vi "Bang Bang Temperature Controller.vi"() -> ()   [LabVIEW 2021]
uses:
  BT.lvlib
  Support/Nodes/Decorators/Repeater/Support/Finish On - Type.ctl
  Support/Nodes/Decorators/Repeater/bt_Repeater.lvclass
  <vilib>/TSA/Omni-Bus/Omni-Bus/Omni_Bus.lvclass
  <vilib>/TSA/Abstract Data Classes/Constants/Support/DBL/DBL.vi
  <vilib>/TSA/Abstract Data Classes/Constants/Support/DBL/Const_DBL.lvclass
  C:/Program Files (x86)/National Instruments/LabVIEW 2021/vi.lib/TSA/Abstract Data Classes/Abs_Types/Double Float/Abs_Double Float.lvclass
  C:/Program Files (x86)/National Instruments/LabVIEW 2021/vi.lib/TSA/Abstract Data Classes/Abs_Types/Floating Point/Abs_Floating Point.lvclass
  C:/Program Files (x86)/National Instruments/LabVIEW 2021/vi.lib/TSA/Abstract Data Classes/Abs_Types/Numeric/Abs_Numeric.lvclass
  C:/Program Files (x86)/National Instruments/LabVIEW 2021/vi.lib/TSA/Abstract Data Classes/Abs_Types/Value/Abs_Value.lvclass
  C:/Program Files (x86)/National Instruments/LabVIEW 2021/vi.lib/TSA/Abstract Data Classes/Abs_Types/Type/Abs_Type.lvclass
  C:/Program Files (x86)/National Instruments/LabVIEW 2021/vi.lib/TSA/Abstract Data Classes/Constants/Support/DBL/Const_DBL.lvclass
  C:/Program Files (x86)/National Instruments/LabVIEW 2021/vi.lib/TSA/Abstract Data Classes/Constants/Support/Interface/Const_Intf.lvclass
  <vilib>/TSA/Omni-Bus/Local Bus/Local Bus.lvclass
  <vilib>/Utility/Data Type/Type Definitions/Data Type.ctl
  <vilib>/Utility/Data Type/NI_Data Type.lvlib
  <vilib>/TSA/Omni-Bus/Local Bus/Support/Tag List Type.ctl
  System/bt_System.lvclass
  <vilib>/TSA/Omni-Bus/Omni-Bus/Support/Get/Get DBL.vi
  <vilib>/TSA/Omni-Bus/Omni-Bus/Support/Get/Get Boolean.vi
  <vilib>/TSA/Omni-Bus/Omni-Bus/Support/Read/Read Boolean.vi
  <vilib>/TSA/Omni-Bus/Omni-Bus/Support/Write/Write DBL.vi
  <vilib>/TSA/Event Log/abs_EventLog/Support/Facility Code.ctl
  <vilib>/TSA/Event Log/abs_EventLog/abs_EventLog.lvclass
  <vilib>/TSA/Event Log/abs_EventLog/Support/Severity Code.ctl
  <vilib>/TSA/Event Log/Event_TextLog/Event_TextLog.lvclass
  C:/Program Files (x86)/National Instruments/LabVIEW 2021/vi.lib/TSA/Omni-Bus/Omni-Bus/Bus Access/Bus_Access.lvclass
  C:/Program Files (x86)/National Instruments/LabVIEW 2021/vi.lib/TSA/Omni-Bus/Local Bus/Local Bus.lvclass
  C:/Program Files (x86)/National Instruments/LabVIEW 2021/vi.lib/TSA/Event Log/abs_EventLog/abs_EventLog.lvclass
  C:/Program Files (x86)/National Instruments/LabVIEW 2021/vi.lib/TSA/Event Log/Event_TextLog/Event_TextLog.lvclass
  Support/Nodes/abs_Node/Status.ctl
  Support/Nodes/abs_Node/bt_Node.lvclass
panel:
  out "Event Messages":string
  out "Status":T1
  out "Waveform Chart":cluster{"Temperature Reading":dbl, i16}(graph)
  in  "stop":bool
  in  "Temperature Reading\n(User Simulated)":dbl(slide) scale=0.0..100.0
  out "Heater":bool
  in  "Hystersis":dbl=2.0
  in  "Temperature Setting":dbl=50.0
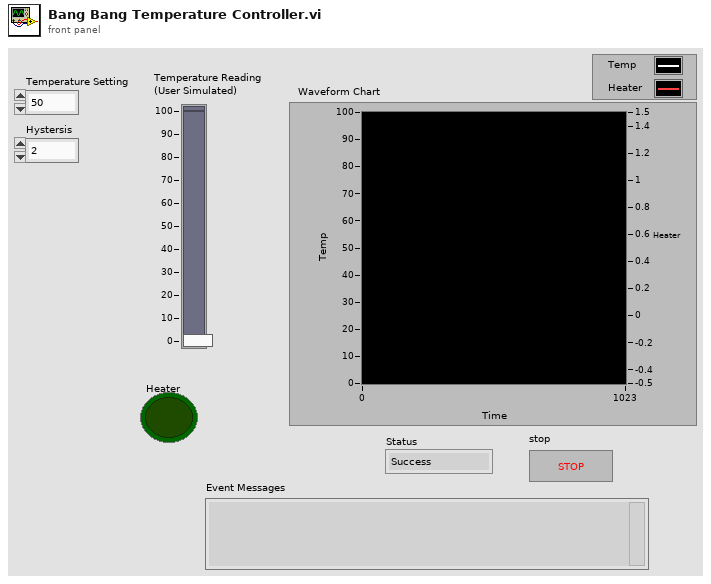
[diagram p1: front panel]
types:
  T1 = typedef "BT.lvlib/bt_Node.lvclass/Status.ctl" = enum16{"Success", "Failure", "Running"}
  T2 = typedef "abs_EventLog.lvclass/Severity Code.ctl" = enum16{"emergency", "alert", "critical", "error", "warning", "notice", "info", "debug"}
  T3 = typedef "abs_EventLog.lvclass/Facility Code.ctl" = enum16{"kernel", "user", "mail", "system daemons", "security/authorization", "syslogd", "line printer", "network news", "uucp", "clock daemon", "security/authorization (alternate)", "FTP daemon", "NTP subsystem", "log audit", "log alert", "clock daemon (alternate)", "local use 0", "local use 1", "local use 2", "local use 3", "local use 4", "local use 5", "local use 6", "local use 7"}
  T4 = typedef "Local Bus.lvclass/Tag List Type.ctl" = cluster{"Tag":string, "Type":T5}
  T5 = typedef "NI_Data Type.lvlib/Data Type.ctl" = enum8{"Invalid Type", "Void", "I8", "I16", "I32", "I64", "U8", "U16", "U32", "U64", "Single Float", "Double Float", "Extended Float", "Single Complex", "Double Complex", "Extended Complex", "Enum U8", "Enum U16", "Enum U32", "Enum U64", "Single Float With Unit", "Double Float With Unit", "Extended Float With Unit", "Single Complex with Unit", "Double Complex with Unit", "Extended Complex with Unit", "Boolean", "String", "Path", "Picture", "Tag", "Array", "Cluster", "Variant", "LV Variant", "Waveform", "Timestamp", "Digital Waveform", "Digital Data", "ExpressData", "Refnum", "External Data", "VI", "Poly VI", "LabVIEW Class Instance", "Fixed Point", "Set Collection", "Map Collection"}
  T6 = typedef "BT.lvlib/bt_Repeater.lvclass/Finish On - Type.ctl" = enum16{"Success", "Failure", "Never"}
  T7 = cluster{"Temperature Reading\n(User Simulated)":dbl, i16}
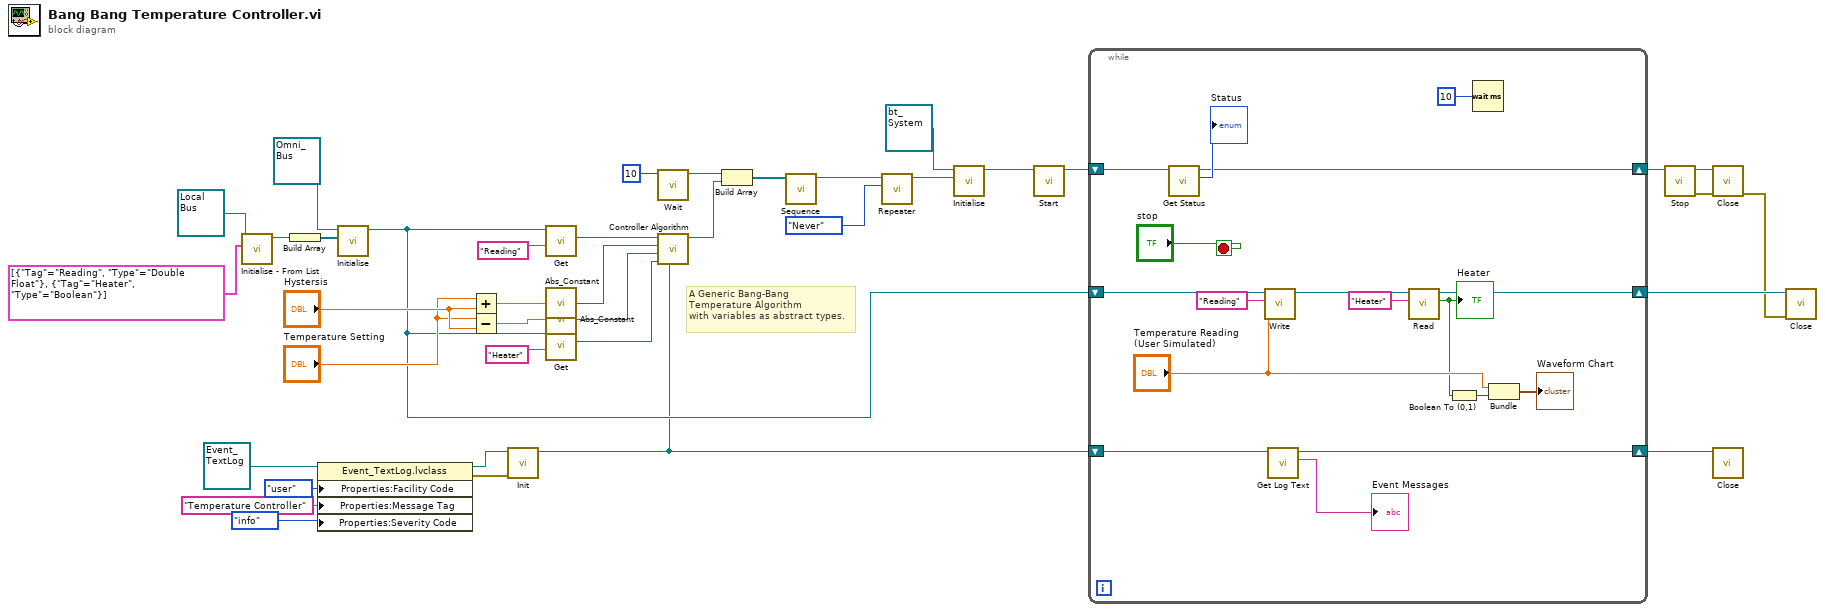
[diagram p0: block diagram]
diagram:
  # "A Generic Bang-Bang \nTemperature Algorithm\nwith variables as abstract types."
  n1 = call <vilib>:"Initialise - From List.vi"("Tag List"=T4[] [{"Tag"="Reading", "Type"=enum."Double Float"}, {"Tag"="Heater", "Type"=enum."Boolean"}], "Local Bus in"=refnum<class "Local Bus.lvclass"> refnum) -> ("Local Bus out"=w21:refnum<class "Local Bus.lvclass">)  [unwired: 8 in, 1 out]
  n2 = Build Array(w21) -> (w22:refnum<class "Local Bus.lvclass">[])
  n3 = property class="Event_TextLog.lvclass"(reference=refnum<class "Event_TextLog.lvclass"> refnum ("Event_TextLog.lvclass"), "Properties:Facility Code"=Facility_Code."user" ("Facility Code"), "Properties:Message Tag"="Temperature Controller" ("Message Tag"), "Properties:Severity Code"=Severity_Code."info" ("Severity Code")) -> (reference out=w3:refnum<class "Event_TextLog.lvclass">, error out=w2:errorcluster)  [unwired: 1 in]
  n4 = call-dynamic "Initialise.vi"("Bus Access"=w22, "Var Bus in"=refnum<class "Omni_Bus.lvclass"> refnum) -> ("Var Bus out"=w19:refnum<class "Omni_Bus.lvclass">)  [unwired: 8 in, 1 out]
  n5 = Add(x="Temperature Setting", y="Hystersis") -> (x+y=w32:dbl)
  n6 = Subtract(x="Temperature Setting", y="Hystersis") -> (x-y=w31:dbl)
  n7 = call-dynamic "Init.vi"("error in (no error)"=w2, "Event_TextLog in"=w3) -> ("Event_TextLog out"=w1:refnum<class "Event_TextLog.lvclass">)  [unwired: 8 in, 1 out]
  n8 = call-poly <vilib>:"Get.vi"("Tag"="Reading", "Var Bus in"=w19) -> ("Value Out"=w38:refnum<class "Abs_Double Float.lvclass">)  [unwired: 6 in, 3 out]
  n9 = call-poly <vilib>:"Abs_Constant.vi"("Value"=w32) -> ("Constant"=w37:refnum<class "Const_DBL.lvclass">)  [unwired: 4 in]
  n10 = call-poly <vilib>:"Abs_Constant.vi"("Value"=w31) -> ("Constant"=w36:refnum<class "Const_DBL.lvclass">)  [unwired: 4 in]
  n11 = call-poly <vilib>:"Get.vi"("Tag"="Heater", "Var Bus in"=w19) -> ("Value Out"=w35:refnum<class "Abs_Boolean.lvclass">)  [unwired: 6 in, 3 out]
  n12 = call "Wait.vi"("Time (ms)"=u32 10) -> ("Node Out"=w26:refnum<class "bt_Node.lvclass">)  [unwired: 10 in]
  n13 = call "Controller Algorithm.vi"("EventLog"=w1, "Heater Output"=w35, "Lower Limit"=w36, "Upper Limit"=w37, "Reading"=w38) -> ("Node Out"=w28:refnum<class "bt_Node.lvclass">)  [unwired: 6 in]
  n14 = Build Array(w26, w28) -> (w27:refnum<class "bt_Node.lvclass">[])
  n15 = call "Sequence.vi"("Nodes"=w27) -> ("Node"=w24:refnum<class "bt_Node.lvclass">)  [unwired: 10 in]
  n16 = call "Repeater.vi"("Finish On"=Finish_On_-_Type."Never", "Node In"=w24) -> ("Node Out"=w10:refnum<class "bt_Node.lvclass">)  [unwired: 9 in]
  n17 = call "Initialise.vi"("Behaviour Tree"=w10, "bt_System in"=refnum<class "bt_System.lvclass"> refnum) -> ("bt_System out"=w11:refnum<class "bt_System.lvclass">)  [unwired: 8 in, 1 out]
  n18 = call "Start.vi"("bt_System in"=w11) -> ("bt_System out"=w15:refnum<class "bt_System.lvclass">)  [unwired: 9 in, 1 out]
  n19 = while {
    shift-right: [w43] -> w14
    shift-left: w15 -> [w46]
    shift-right: [w54] -> w17
    shift-left: w19 -> [w56]
    shift-right: [w41] -> w4
    shift-left: w1 -> [w42]
    stop <- "stop" stop-if-true
    n20 = call "Get Status.vi"("bt_System in"=w46) -> ("Status"=→"Status":T1, "bt_System out"=w43:refnum<class "bt_System.lvclass">)  [unwired: 8 in, 1 out]
    n21 = call-poly <vilib>:"Write.vi"("Numeric"="Temperature Reading\n(User Simulated)", "Tag"="Reading", "Omni_Bus in"=w56) -> ("Omni_Bus out"=w55:refnum<class "Omni_Bus.lvclass">)  [unwired: 7 in, 1 out]
    n22 = call <vilib>:"Get Log Text.vi"("Event_TextLog in"=w42) -> ("Log Message"=→"Event Messages":string, "Event_TextLog out"=w41:refnum<class "Event_TextLog.lvclass">)  [unwired: 8 in, 1 out]
    n23 = call-poly <vilib>:"Read.vi"("Tag"="Heater", "Var Bus in"=w55) -> ("Boolean"=w49:bool, "Var Bus out"=w54:refnum<class "Omni_Bus.lvclass">)  [unwired: 7 in, 1 out]
    "Heater" <- w49
    n24 = Boolean To (0,1)(Boolean=w49) -> (0, 1=w50:i16)
    n25 = Wait (ms)(milliseconds to wait=u32 10) -> ()  [unwired: 1 out]
    n26 = Bundle("Temperature Reading\n(User Simulated)"="Temperature Reading\n(User Simulated)", w50) -> (→"Waveform Chart":T7)  [unwired: 1 in]
  }
  n27 = call "Stop.vi"("bt_System in"=w14) -> ("error out"=w12:errorcluster, "bt_System out"=w13:refnum<class "bt_System.lvclass">)  [unwired: 9 in]
  n28 = call-dynamic "Close.vi"("error in (no error)"=w12, "bt_System in"=w13) -> ("error out"=w16:errorcluster)  [unwired: 8 in, 1 out]
  n29 = call-dynamic "Close.vi"("Event_TextLog in"=w4) -> ()  [unwired: 9 in, 2 out]
  n30 = call-dynamic "Close.vi"("error in (no error)"=w16, "Data in"=w17) -> ()  [unwired: 8 in, 2 out]
